vi "SLL DE DO Response LV2Global.vi"(6 "Option":T1=enum."Send Response", 8 "Error in (no error)":errorcluster, 11 "Executed For?":string) -> (0 "Error out":errorcluster, 3 "Found?":bool)   [LabVIEW 2013]
uses:
  Controls/SLL DE DO Response LV2Global Options.ctl
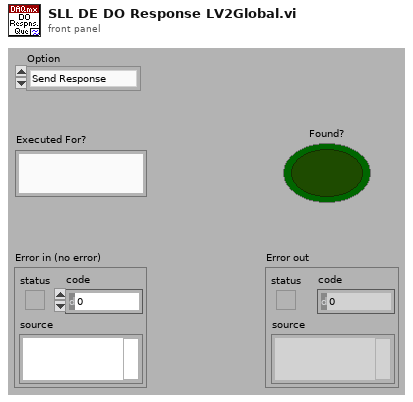
[diagram p1: front panel]
types:
  T1 = typedef "SLL DE DO Response LV2Global Options.ctl" = enum16{"Initialize", "Send Response", "Check Response", "Close"}
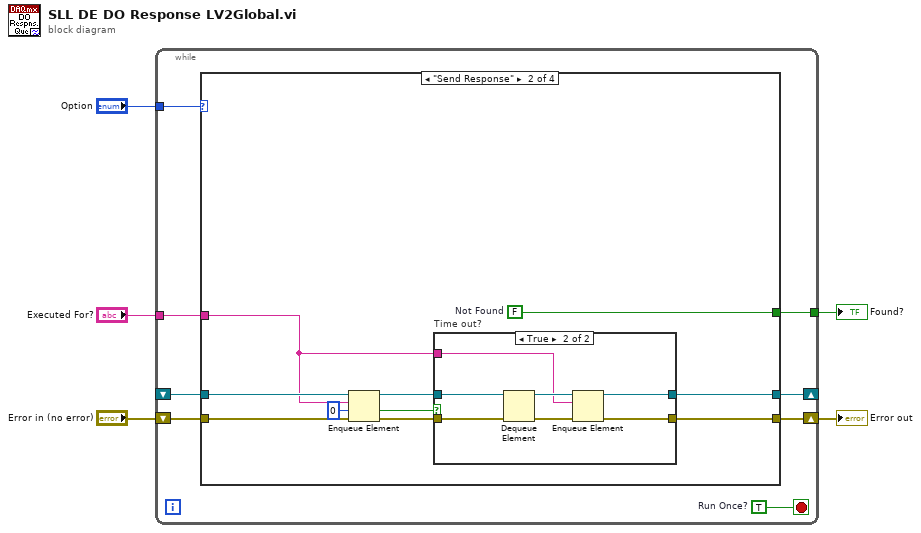
[diagram p0: block diagram]
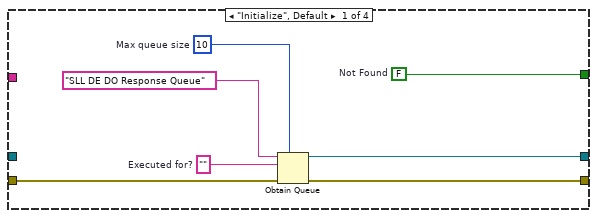
[diagram p2: hidden frame]
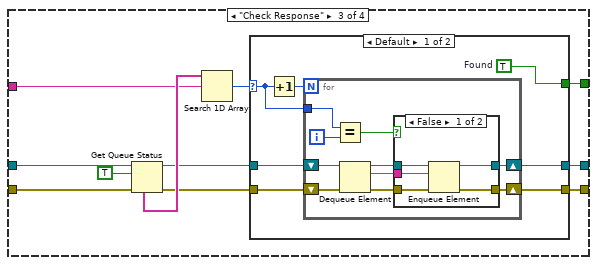
[diagram p4: hidden frame]
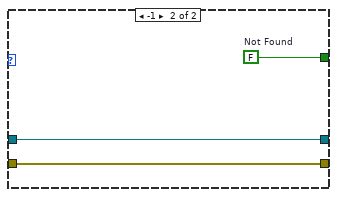
[diagram p6: hidden frame]
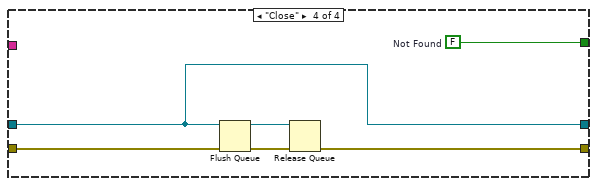
[diagram p7: hidden frame]
diagram:
  n1 = while {
    tunnel: "Option" -> [w12]
    shift-right: [w11] -> _
    shift-left: _ -> [w10]
    tunnel: "Executed For?" -> [w9]
    shift-right: [w7] -> w2
    shift-left: "Error in (no error)" -> [w8]
    tunnel: [w6] -> w1
    stop <- w13 stop-if-true
    w13 = TRUE  # Run Once?
    n2 = case shown="\"Send Response\"" w12 {
      tunnel: [w16 w21 w42 w80] -> w11
      tunnel: w10 -> [_ w30 w49 w80]
      tunnel: w9 -> [_ w25 w46 _]
      tunnel: w8 -> [w18 w29 w50 w81]
      tunnel: [w17 w22 w41 w79] -> w7
      tunnel: [w14 w28 w40 w78] -> w6
      frame "Initialize", Default {
        w14 = FALSE  # Not Found
        w15 = 10  # Max queue size
        w19 = ""  # Executed for?
        n3 = Obtain Queue(max queue size (-1, unlimited)=w15, name (unnamed)="SLL DE DO Response Queue", element data type=w19, error in (no error)=w18) -> (queue out=w16:refnum<queue>, error out=w17:errorcluster)  [unwired: 1 in, 1 out]
      }
      frame "Send Response" {
        w28 = FALSE  # Not Found
        n4 = Enqueue Element(queue=w30, element=w25, timeout in ms (-1)=0, error in (no error)=w29) -> (queue out=w26:refnum<queue>, timed out?=w24:bool, error out=w27:errorcluster)
        n5 = case "Time out?" shown="True" w24 {
          tunnel: w27 -> [w32 w38]
          tunnel: w26 -> [w31 w39]
          tunnel: [w32 w36] -> w22
          tunnel: [w31 w35] -> w21
          tunnel: w25 -> [_ w33]
          frame False {
          }
          frame True {
            n6 = Dequeue Element(queue=w39, error in (no error)=w38) -> (queue out=w34:refnum<queue>, error out=w37:errorcluster)  [unwired: 1 in, 2 out]
            n7 = Enqueue Element(queue=w34, element=w33, error in (no error)=w37) -> (queue out=w35:refnum<queue>, error out=w36:errorcluster)  [unwired: 1 in, 1 out]
          }
        }
      }
      frame "Check Response" {
        n8 = Get Queue Status(queue=w49, return elements? (F)=TRUE, error in (no error)=w50) -> (queue out=w44:refnum<queue>, error out=w43:errorcluster, elements=w47:string[])  [unwired: 5 out]
        n9 = Search 1D Array(1D array=w47, element=w46) -> (index of element=w45:i32)  [unwired: 1 in]
        n10 = case shown="Default" w45 {
          selector: w45 -> [w51 _]
          tunnel: w44 -> [w54 w77]
          tunnel: w43 -> [w57 w76]
          tunnel: [w56 w77] -> w42
          tunnel: [w55 w76] -> w41
          tunnel: [w53 w75] -> w40
          frame Default {
            w53 = TRUE  # Found
            n11 = Increment(x=w51) -> (x+1=w52:i32)
            n12 = for {
              N: w52 -> [_]
              shift-right: [w60] -> w56
              shift-left: w54 -> [w66]
              shift-right: [w59] -> w55
              shift-left: w57 -> [w67]
              tunnel: w51 -> [w64]
              i -> [w65]
              n13 = Equal?(x=w64, y=w65) -> (x = y?=w63:bool)
              n14 = Dequeue Element(queue=w66, error in (no error)=w67) -> (queue out=w61:refnum<queue>, element=w58:string, error out=w62:errorcluster)  [unwired: 1 in, 1 out]
              n15 = case shown="False" w63 {
                tunnel: w62 -> [w72 w73]
                tunnel: w61 -> [w71 w74]
                tunnel: [w70 w74] -> w60
                tunnel: [w69 w73] -> w59
                tunnel: w58 -> [w68 _]
                frame False {
                  n16 = Enqueue Element(queue=w71, element=w68, error in (no error)=w72) -> (queue out=w70:refnum<queue>, error out=w69:errorcluster)  [unwired: 1 in, 1 out]
                }
                frame True {
                }
              }
            }
          }
          frame -1 {
            w75 = FALSE  # Not Found
          }
        }
      }
      frame "Close" {
        w78 = FALSE  # Not Found
        n17 = Flush Queue(queue=w80, error in (no error)=w81) -> (queue out=w83:refnum<queue>, error out=w82:errorcluster)  [unwired: 1 out]
        n18 = Release Queue(queue=w83, error in (no error)=w82) -> (error out=w79:errorcluster)  [unwired: 1 in, 2 out]
      }
    }
  }
  "Error out" <- w2
  "Found?" <- w1
